vi "frequency estimation my computer.vi"() -> ()   [LabVIEW 2014]
uses:
  <vilib>/FPGAPlugInAG/cRIO-9063/niLvFpga_Open_cRIO-9063.vi
  <vilib>/rvi/interface/common/dynamic/niFpgaDynamicAddResources.vi
  <vilib>/Utility/error.llb/Error Cluster From Error Code.vi
  <vilib>/rvi/errors/niLvFpgaAdjustHostInterfaceError.vi
  <vilib>/FPGAPlugInAG/Dynamic/niLvFpga_Close_Dynamic.vi
  <vilib>/rvi/interface/nirviOpenFPGA/nirviOpenFPGA.xnode
  Projects/FPGA Bitfiles/frequencyestimat_FPGATarget_frequencyestimat_QVNc5bBiVHY.lvbitx
  frequency estimation special.vi
  <vilib>/rvi/interface/nirviMethod/nirviMethod.xnode
  <vilib>/rvi/interface/nirviCloseFPGA/nirviCloseFPGA.xnode
  <vilib>/FPGAPlugInAG/Dynamic/niLvFpga_ReadFifo_Dynamic.vi
  <vilib>/rvi/errors/niLvFpgaMergeErrorWithErrorCode.vi
panel:
  out "del f)":dbl
  out "Frequency":dbl
  out "a":cdb
  out "element 3":fxp<+/-,25,11>
  out "element 2":fxp<+/-,25,11>
  out "element":fxp<+/-,25,11>
  out "decimated array 3":fxp<+/-,25,11>[](array[numeric])
  out "decimated array 2":fxp<+/-,25,11>[](array[numeric])
  out "decimated array":fxp<+/-,25,11>[](array[numeric])
  out "Angle \nElements Remaining":u32
  out "Angles":fxp<+/-,16,16>[](array[numeric])
  out "magnitude\nElements Remaining":u32
  out "magnitude":fxp<+/-,25,11>[](array[numeric])
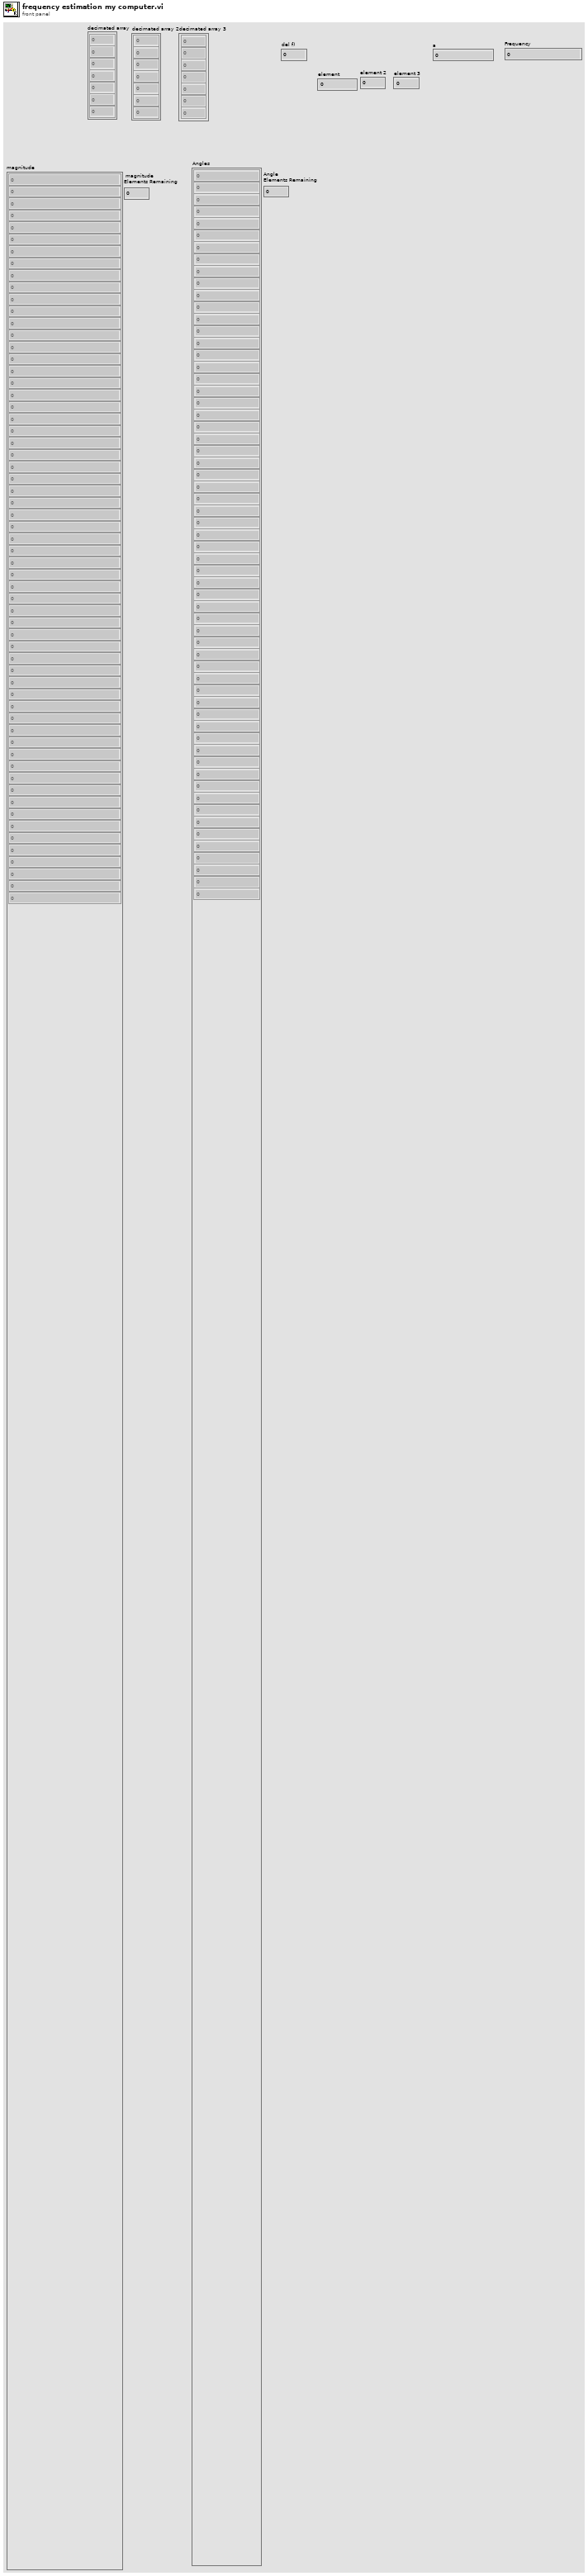
[diagram p1: front panel]
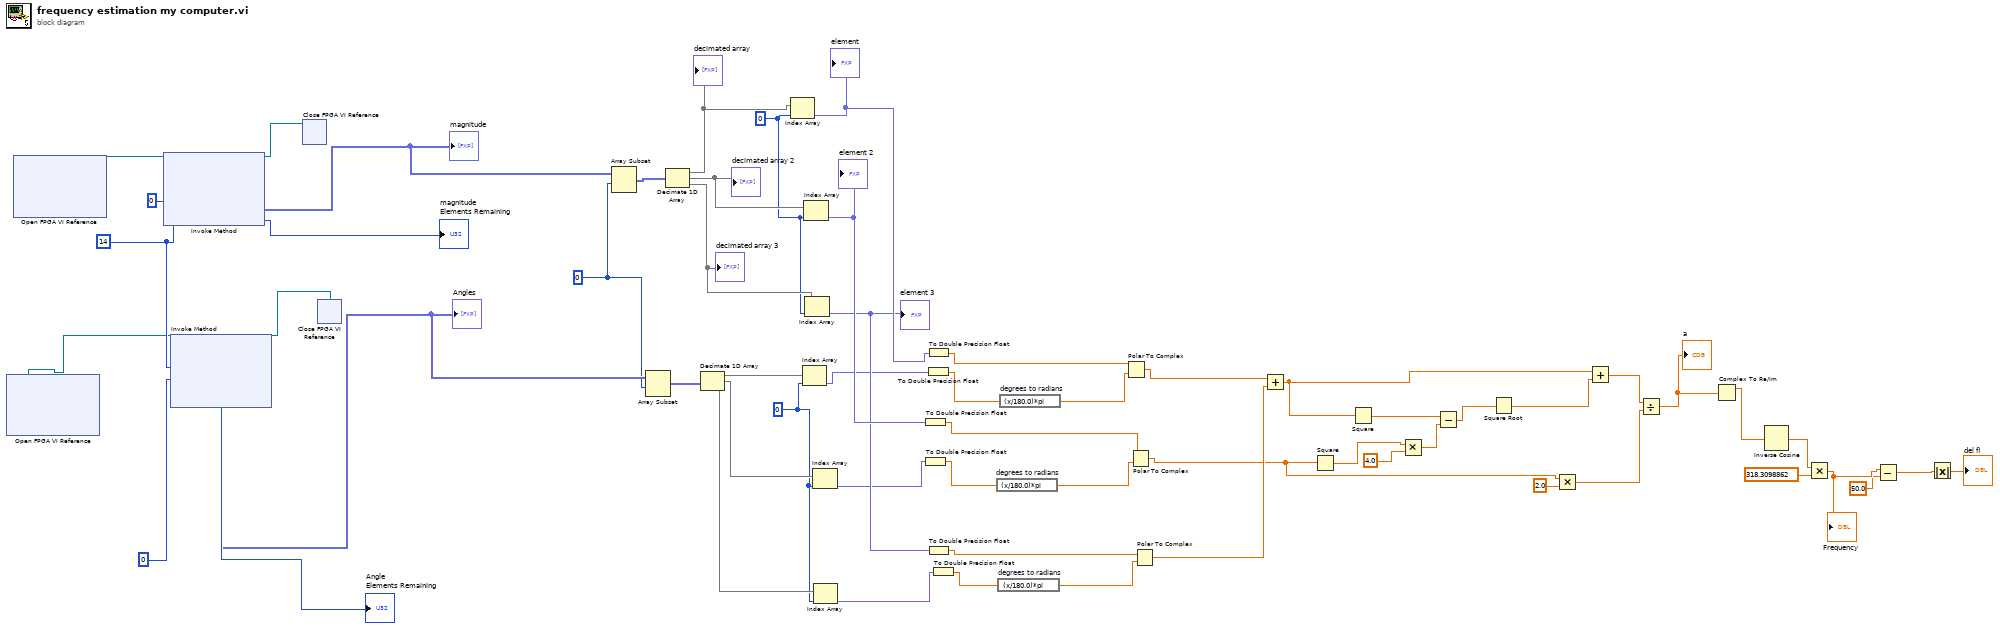
[diagram p0: block diagram]
diagram:
  w5 = 0 ("index")
  w23 = 0 ("index")
  w42 = 0 ("index")
  w51 = u32 14 ("Number of Elements")
  n1 = xnode "Open FPGA VI Reference"() -> ("FPGA VI Reference Out"=w49:refnum<k20>)  [unwired: 2 in, 1 out]
  n2 = xnode "Open FPGA VI Reference"() -> ("FPGA VI Reference Out"=w50:refnum<k20>)  [unwired: 2 in, 1 out]
  n3 = xnode "Invoke Method"("FPGA VI Reference In"=w50, "Number of Elements"=w51, "Timeout (ms)"=0) -> ("FPGA VI Reference Out"=w57:refnum<k20>, "Data"=w52:fxp<+/-,25,11>[], "Elements Remaining"=→"magnitude\nElements Remaining":u32)  [unwired: 1 in, 1 out]
  "magnitude" <- w52
  n4 = xnode "Invoke Method"("FPGA VI Reference In"=w49, "Number of Elements"=w51, "Timeout (ms)"=0) -> ("FPGA VI Reference Out"=w55:refnum<k20>, "Data"=w48:fxp<+/-,16,16>[], "Elements Remaining"=→"Angle \nElements Remaining":u32)  [unwired: 1 in, 1 out]
  "Angles" <- w48
  n5 = xnode "Close FPGA VI Reference"("FPGA VI Reference In"=w57) -> ()  [unwired: 1 in, 1 out]
  n6 = xnode "Close FPGA VI Reference"("FPGA VI Reference In"=w55) -> ()  [unwired: 1 in, 1 out]
  n7 = Array Subset(array=w52, index=w5) -> (w47:fxp<+/-,25,11>[])  [unwired: 1 in]
  n8 = Array Subset(array=w48, index=w5) -> (w46:fxp<+/-,16,16>[])  [unwired: 1 in]
  n9 = Decimate 1D Array(w47) -> (w45:fxp<+/-,25,11>[], w44:fxp<+/-,25,11>[], w43:fxp<+/-,25,11>[])
  "decimated array" <- w45
  "decimated array 2" <- w44
  "decimated array 3" <- w43
  n10 = Decimate 1D Array(w46) -> (w35:fxp<+/-,16,16>[], w34:fxp<+/-,16,16>[], w33:fxp<+/-,16,16>[])
  n11 = Index Array(array=w45, index=w42) -> (element=w32:fxp<+/-,25,11>)
  "element" <- w32
  n12 = Index Array(array=w35, index=w23) -> (element=w26:fxp<+/-,16,16>)
  n13 = Index Array(array=w44, index=w42) -> (element=w30:fxp<+/-,25,11>)
  "element 2" <- w30
  n14 = Index Array(array=w43, index=w42) -> (element=w28:fxp<+/-,25,11>)
  "element 3" <- w28
  n15 = Index Array(array=w34, index=w23) -> (element=w25:fxp<+/-,16,16>)
  n16 = Index Array(array=w33, index=w23) -> (element=w24:fxp<+/-,16,16>)
  n17 = To Double Precision Float(number=w30) -> (double precision float=w29:dbl)
  n18 = To Double Precision Float(number=w25) -> (double precision float=w9:dbl)
  n19 = To Double Precision Float(number=w26) -> (double precision float=w11:dbl)
  n20 = To Double Precision Float(number=w32) -> (double precision float=w31:dbl)
  n21 = To Double Precision Float(number=w28) -> (double precision float=w27:dbl)
  n22 = To Double Precision Float(number=w24) -> (double precision float=w7:dbl)
  n23 = expression code="(x/180.0)*pi" "degrees to radians"(w9) -> (w8:dbl)
  n24 = expression code="(x/180.0)*pi" "degrees to radians"(w7) -> (w6:dbl)
  n25 = expression code="(x/180.0)*pi" "degrees to radians"(w11) -> (w10:dbl)
  n26 = Polar To Complex(1:w10, 2:w31) -> (0:w22:cdb)
  n27 = Polar To Complex(1:w8, 2:w29) -> (0:w17:cdb)
  n28 = Polar To Complex(1:w6, 2:w27) -> (0:w21:cdb)
  n29 = Add(x=w22, y=w21) -> (x+y=w41:cdb)
  n30 = Square(x=w17) -> (x^2=w38:cdb)
  n31 = Square(x=w41) -> (x^2=w40:cdb)
  n32 = Multiply(x=w38, y=4.0) -> (x*y=w37:cdb)
  n33 = Subtract(x=w40, y=w37) -> (x-y=w36:cdb)
  n34 = Square Root(x=w36) -> (sqrt(x)=w20:cdb)
  n35 = Multiply(x=w17, y=2.0) -> (x*y=w16:cdb)
  n36 = Add(x=w41, y=w20) -> (x+y=w19:cdb)
  n37 = Divide(x=w19, y=w16) -> (x/y=w15:cdb)
  "a" <- w15
  n38 = Complex To Re/Im(x + iy=w15) -> (x=w14:dbl)  [unwired: 1 out]
  n39 = Inverse Cosine(1:w14) -> (0:w13:dbl)
  n40 = Multiply(x=w13, y=318.3098862) -> (x*y=w4:dbl)
  "Frequency" <- w4
  n41 = Subtract(x=w4, y=50.0) -> (x-y=w2:dbl)
  n42 = Absolute Value(x=w2) -> (abs(x)=→"del f)":dbl)
